vi "image_recording.vi"() -> ()   [LabVIEW 2011]
uses:
  <vilib>/userdefined/High Color/IMAQdx.ctl
  global_vars.vi
  <vilib>/vision/driver/NI_Vision_Acquisition_Software.lvlib
  C:/Program Files/National Instruments/LabVIEW 2011/resource/objmgr/imaqdx.rc
panel:
  out "selected image":T1(plugin-control)
  in  "dbl_ar_#fringes":dbl[](array[numeric])=[5.0]
  out "u8_ar_cur_sel_fringe#_dist":u8[][][](array[numeric])
  out "u8_ar_cur_sel_fringe#_orig":u8[][][](array[numeric])
  in  "phase shift":i32=3
  in  "dist/orig":u16(ring)=1 items=["original", "distorted"]
  in  "direction":u16(ring) items=["x-direction", "y-direction"]
  out "dbl_sel_#fringes":dbl=5.0
  in  "measurement":i32
  out "u8_ar_all_images":u8[][][][][][](array[numeric])
  in  "start align":bool
  in  "b_default prefix":bool=TRUE
  in  "b_save_orig":bool=TRUE caption="original"
  in  "b_save_captured":bool caption="captured"
  in  "image prefix":string
  out "b_meas_running":bool caption="Measurement\nRunning"
  in  "df_intial phase shift":dbl
  in  "UL_#Phase Shifts":i32=4
  out "p_experiment_path":path=path "X:/Cloud Drives/Dropbox/Europhotonics/FringeMan/Image Storage/02_01"
  in  "EXP File Path 2":path=path "X:/Cloud Drives/Dropbox/Europhotonics/FringeMan/Image Storage" caption="Enter or select file path"
  in  "b_save images":bool caption="save images"
  in  "b_start_meas":bool
  in  "Stop Button":bool
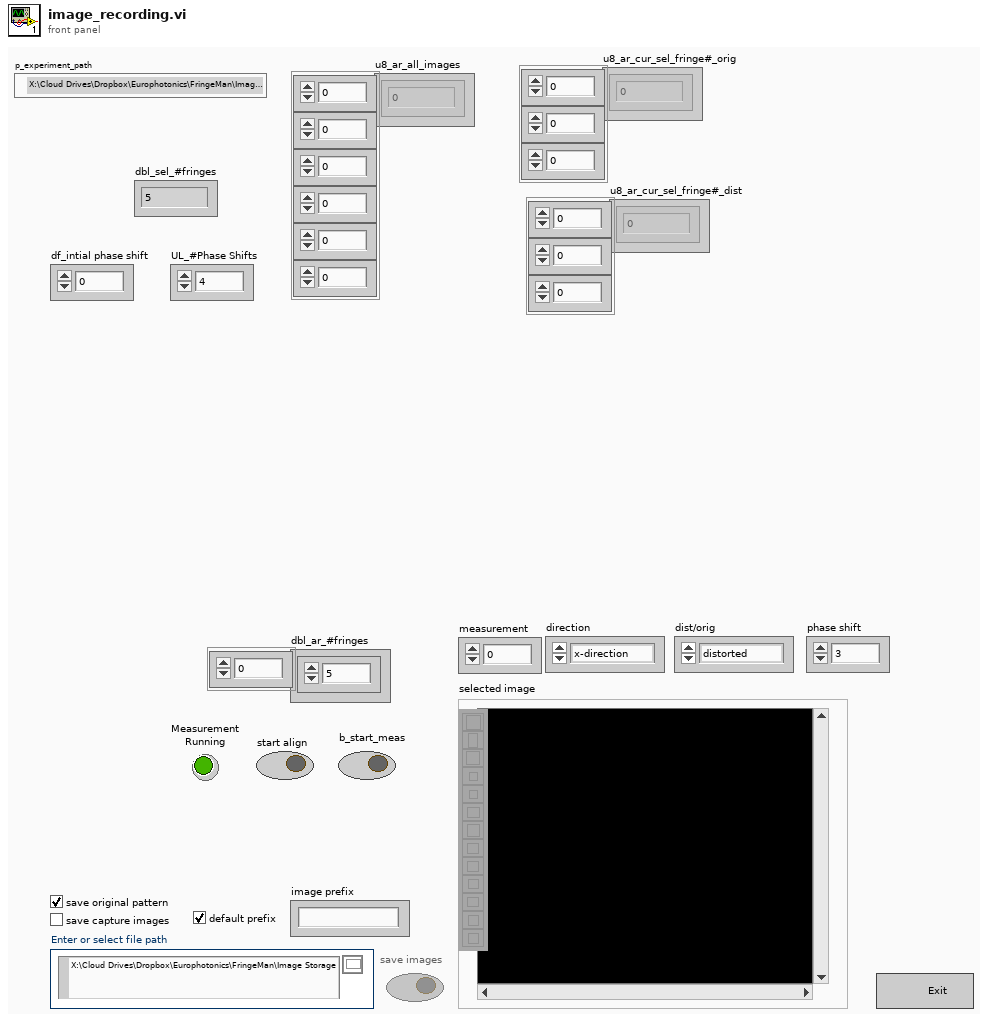
[diagram p1: front panel]
types:
  T1 = typedef "IMAQ Image.ctl" = refnum<image>
  T2 = typedef "IMAQdx.ctl" = refnum<k21>
  T3 = enum8{"Enabled", "Disabled", "Disabled and Grayed Out"}
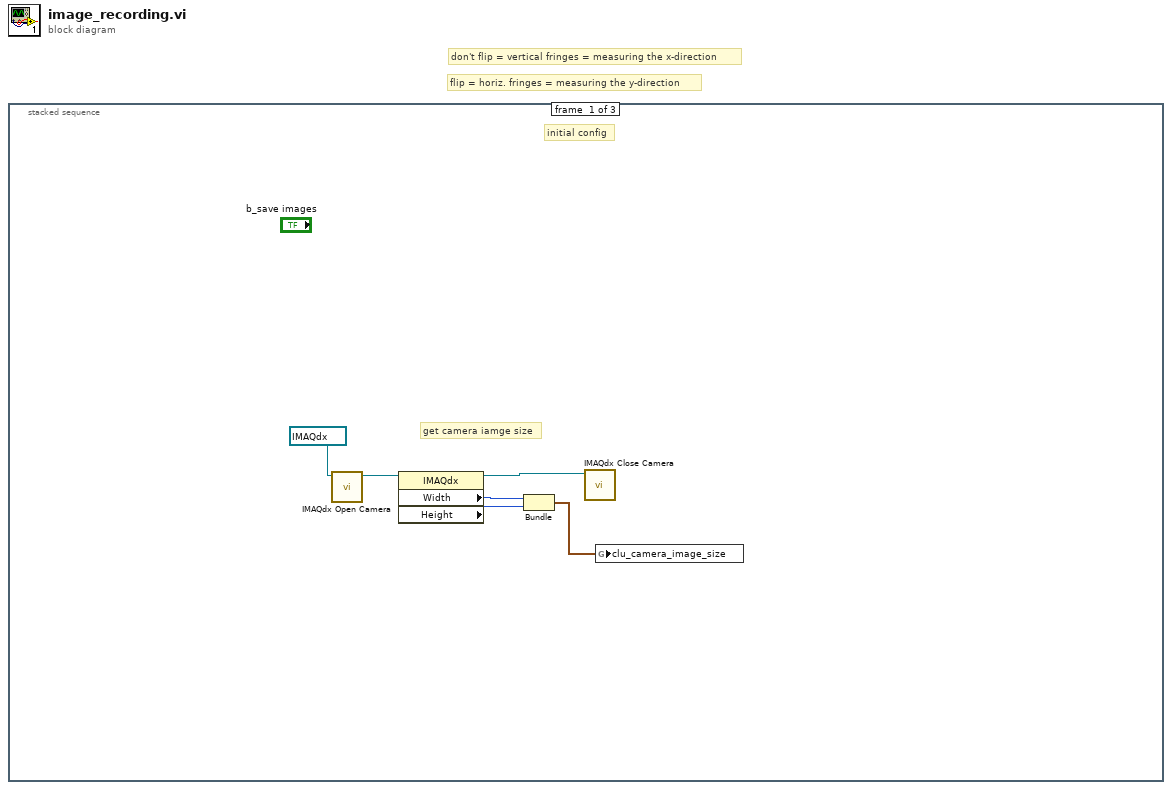
[diagram p0: block diagram]
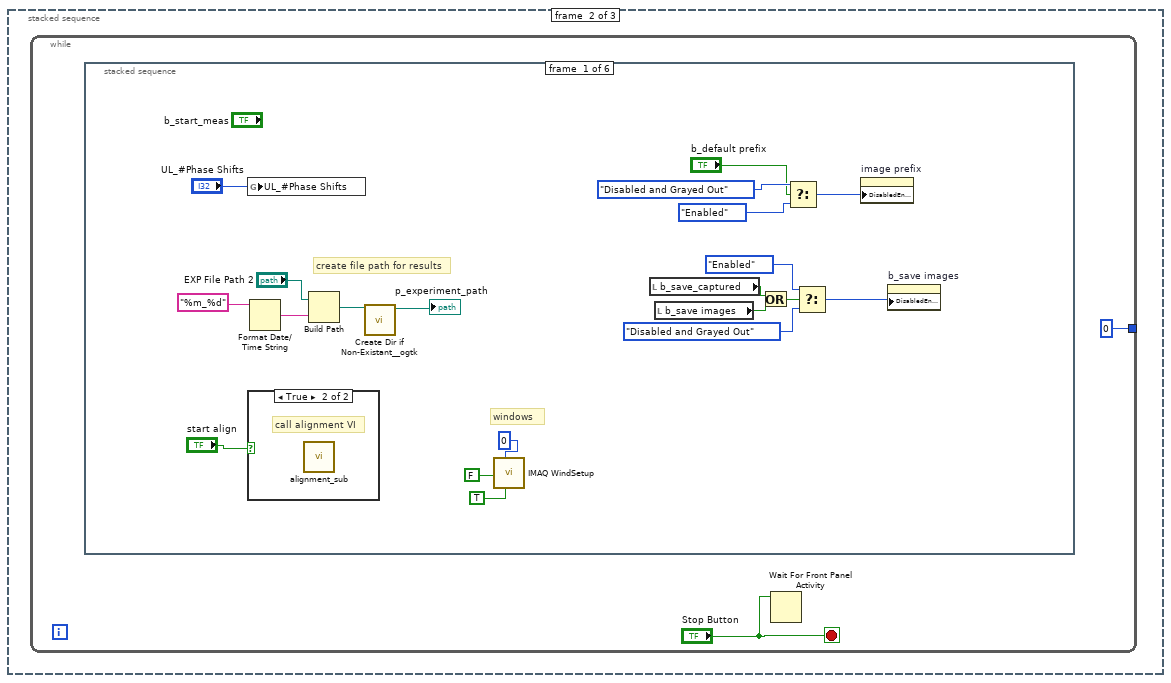
[diagram p2: hidden frame]
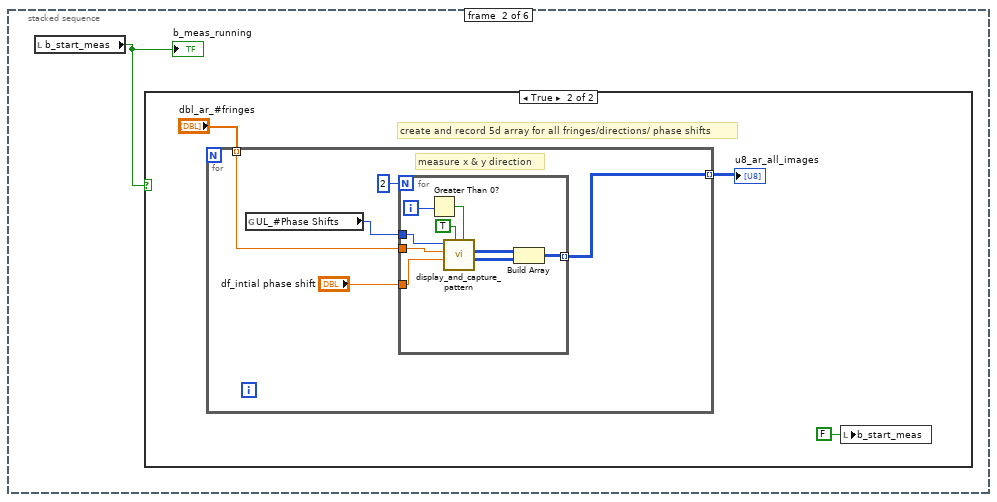
[diagram p4: hidden frame]
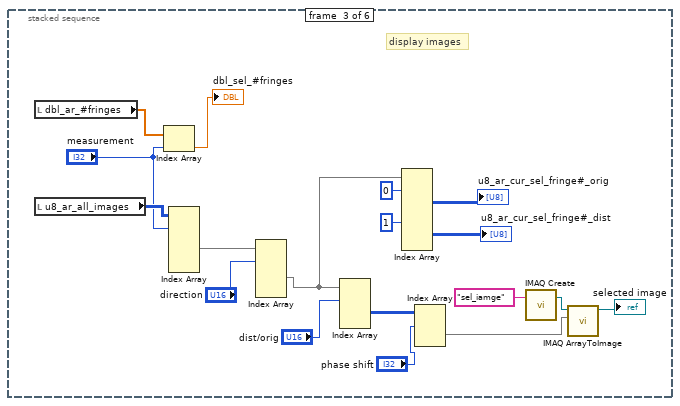
[diagram p6: hidden frame]
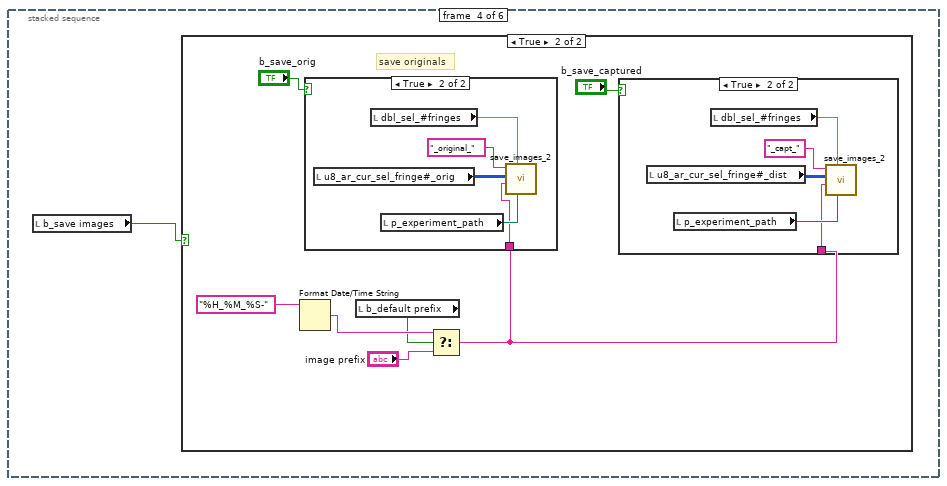
[diagram p7: hidden frame]
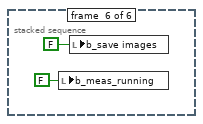
[diagram p12: hidden frame]
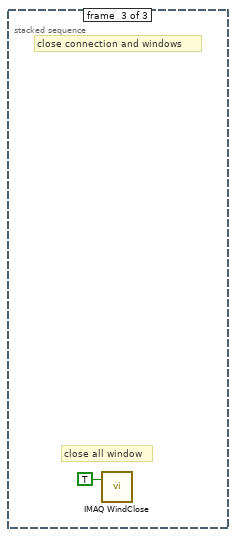
[diagram p13: hidden frame]
diagram:
  # "flip = horiz. fringes = measuring the y-direction"
  # "don't flip = vertical fringes = measuring the x-direction"
  n1 = stacked-sequence {
    frame #0 {
      # "get camera iamge size"
      # "initial config"
      n2 = call <vilib>:"IMAQdx Open Camera.vi"("Session In"=T2 "cam0") -> ("Session Out"=w5:T2)  [unwired: 9 in, 1 out]
      n3 = property class="IMAQdx"(reference=w5) -> (reference out=w4:T2, "Width"=w3:u32, "Height"=w2:u32)  [unwired: 1 in, 1 out]
      n4 = Bundle ("camera_image_size")("Width"=w3, "Height"=w2) -> (w1:cluster{"Width":u32, "Height":u32})  [unwired: 1 in]
      n5 = call <vilib>:"IMAQdx Close Camera.vi"("Session In"=w4) -> ()  [unwired: 10 in, 1 out]
      n6 = global write "global_vars.vi" "clu_camera_image_size"(w1) -> ()
    }
    frame #1 {
      n7 = while {
        tunnel: [0] -> _
        stop <- "Stop Button" stop-if-true
        n8 = stacked-sequence {
          frame #0 {
            # "windows"
            # "create file path for results"
            n9 = global write "global_vars.vi" "UL_#Phase Shifts"("UL_#Phase Shifts") -> ()
            n10 = case shown="True" "start align" {
              frame False {
              }
              frame True {
                # "call alignment VI"
                n11 = call "alignment_sub.vi"() -> ()  [unwired: 12 in]
              }
            }
            n12 = Format Date/Time String(time format string (%c)="%m_%d") -> (date/time string=w25:string)  [unwired: 2 in]
            n13 = Build Path(base path="EXP File Path 2", name or relative path=w25) -> (appended path=w24:path)
            n14 = call <userlib>:"Create Dir if Non-Existant__ogtk.vi"("Directory Path"=w24) -> ("dup Directory Path"=→"p_experiment_path":path)  [unwired: 8 in, 2 out]
            n15 = call "IMAQ WindSetup"("Window is floating? (No)"=TRUE, "Window Number (0...15)"=0, "Window has title bar? (Yes)"=FALSE) -> ()  [unwired: 8 in, 1 out]
            n16 = local read "b_save_captured"() -> (w18:bool)
            n17 = local read "b_save images"() -> (w17:bool)
            n18 = Or(x=w18, y=w17) -> (x .or. y?=w16:bool)
            n19 = Select(t=T3."Disabled and Grayed Out" ("Disabled"), s="b_default prefix", f=T3."Enabled" ("Disabled")) -> (s? t:f=w19:T3)
            n20 = Select(t=T3."Enabled" ("Disabled"), s=w16, f=T3."Disabled and Grayed Out" ("Disabled")) -> (s? t:f=w13:T3)
            n21 = property on="image prefix" class="Str"("DisabledEnum"=w19) -> ()  [unwired: 2 in, 2 out]
            n22 = property on="b_save images" class="Bool (strict)"("DisabledEnum"=w13) -> ()  [unwired: 2 in, 2 out]
          }
          frame #1 {
            n23 = local read "b_start_meas"() -> (w29:bool)
            "b_meas_running" <- w29
            n24 = case shown="True" w29 {
              frame False {
              }
              frame True {
                # "create and record 5d array for all fringes/directions/ phase shifts"
                n25 = for {
                  tunnel: "dbl_ar_#fringes" -> [w36] mode=indexing
                  tunnel: [w34] -> w32 mode=indexing
                  # "measure x & y direction"
                  n26 = global read "global_vars.vi" "UL_#Phase Shifts"() -> (w33:i32)
                  n27 = for {
                    N: 2 -> [_]
                    tunnel: w36 -> [w46]
                    tunnel: "df_intial phase shift" -> [w45]
                    tunnel: [w42] -> w34 mode=indexing
                    tunnel: w33 -> [w38]
                    i -> [w44]
                    n28 = Greater Than 0?(x=w44) -> (x > 0?=w43:bool)
                    n29 = call "display_and_capture_pattern.vi"("flip direction"=w43, "capture images ?"=TRUE ("b_record images"), "intial phase shift"=w45, "#fringes"=w46, "#Phase Shifts"=w38) -> ("ul_ar_pxar_capt_images"=w40:u8[][][], "ul_ar_pxar_orig_pattern"=w41:u8[][][])  [unwired: 5 in]
                    n30 = Build Array(w41, w40) -> (w42:u8[][][][])
                  }
                }
                "u8_ar_all_images" <- w32
                n31 = local write "b_start_meas"(FALSE ("b_start_meas")) -> ()
              }
            }
          }
          frame #2 {
            # "display images"
            n32 = local read "dbl_ar_#fringes"() -> (w64:dbl[])
            n33 = local read "u8_ar_all_images"() -> (w62:u8[][][][][][])
            n34 = Index Array(array=w64, index="measurement") -> (element=→"dbl_sel_#fringes":dbl)
            n35 = Index Array(array=w62, index (dim 0)="measurement") -> (element=w61:u8[][][][][])  [unwired: 5 in]
            n36 = Index Array(array=w61, index (dim 0)="direction") -> (element=w51:u8[][][][])  [unwired: 4 in]
            n37 = Index Array(array=w51, index (dim 0)="dist/orig") -> (element=w48:u8[][][])  [unwired: 3 in]
            n38 = Index Array(array=w51, index (dim 0) #1=0 ("index (vol)"), index (dim 0) #2=1 ("index (vol)")) -> (element #1=→"u8_ar_cur_sel_fringe#_orig":u8[][][], element #2=→"u8_ar_cur_sel_fringe#_dist":u8[][][])  [unwired: 6 in]
            n39 = Index Array(array=w48, index (dim 0)="phase shift") -> (element=w56:u8[][])  [unwired: 2 in]
            n40 = call "IMAQ Create"("Image Name"="sel_iamge" ("current image 3")) -> ("New Image"=w57:T1)  [unwired: 3 in, 2 out]
            n41 = call "IMAQ ArrayToImage"("Image Pixels (U8)"=w56, "Image"=w57) -> ("Image Out"=→"selected image":T1)  [unwired: 8 in, 1 out]
          }
          frame #3 {
            n42 = local read "b_save images"() -> (w65:bool)
            n43 = case shown="True" w65 {
              frame False {
              }
              frame True {
                # "save originals"
                n44 = Format Date/Time String(time format string (%c)="%H_%M_%S-") -> (date/time string=w71:string)  [unwired: 2 in]
                n45 = local read "b_default prefix"() -> (w66:bool)
                n46 = Select(t=w71, s=w66, f="image prefix") -> (s? t:f=w69:string)
                n47 = case shown="True" "b_save_orig" {
                  tunnel: w69 -> [_ w80]
                  frame False {
                  }
                  frame True {
                    n48 = local read "u8_ar_cur_sel_fringe#_orig"() -> (w78:u8[][][])
                    n49 = local read "dbl_sel_#fringes"() -> (w79:dbl)
                    n50 = local read "p_experiment_path"() -> (w82:path)
                    n51 = call "save_images_2.vi"("p_experiment_path"=w82, "number of fringes"=w79, "time (or other uniqe identifier)"=w80, "images to store (3D pixel array)"=w78, "description (orig./capt.)"="_original_") -> ()  [unwired: 7 in]
                  }
                }
                n52 = case shown="True" "b_save_captured" {
                  tunnel: w69 -> [_ w75]
                  frame False {
                  }
                  frame True {
                    n53 = local read "u8_ar_cur_sel_fringe#_dist"() -> (w73:u8[][][])
                    n54 = local read "p_experiment_path"() -> (w77:path)
                    n55 = local read "dbl_sel_#fringes"() -> (w74:dbl)
                    n56 = call "save_images_2.vi"("p_experiment_path"=w77, "number of fringes"=w74, "time (or other uniqe identifier)"=w75, "images to store (3D pixel array)"=w73, "description (orig./capt.)"="_capt_") -> ()  [unwired: 7 in]
                  }
                }
              }
            }
          }
          frame #4 {
            # "this is all yours ccquiel"
            # "calc. phase maps"
          }
          frame #5 {
            n57 = local write "b_meas_running"(FALSE ("b_meas_running")) -> ()
            n58 = local write "b_save images"(FALSE ("b_save images")) -> ()
          }
        }
        n59 = Wait For Front Panel Activity(3:"Stop Button") -> ()  [unwired: 2 in, 1 out]
      }
    }
    frame #2 {
      # "close all window"
      # "close connection and windows"
      n60 = call "IMAQ WindClose"("Close All Windows (False)"=TRUE) -> ()  [unwired: 5 in, 1 out]
    }
  }
